vi "drive_robot.vi"(9 "steering frame velocity":dbl[](array[numeric]), 10 "starter kit differential steering frame":refnum<class "NI_Robotics_Differential Steering Frame.lvclass">, 11 "NI_Robotics_Starter Kit Host_Sim_2.0 in":refnum<class "NI_Robotics_Starter Kit Host_Sim_2.0.lvclass">) -> (3 "NI_Robotics_Starter Kit Host_Sim_2.0 out":refnum<class "NI_Robotics_Starter Kit Host_Sim_2.0.lvclass">)   [LabVIEW 2016]
uses:
  <vilib>/robotics/Starter Kit/2.0/Sim Host Interface/NI_Robotics_Starter Kit Host_Sim_2.0.lvclass
  C:/Program Files (x86)/National Instruments/LabVIEW 2016/vi.lib/robotics/Starter Kit/Host Interface/NI_Robotics_Starter Kit Host.lvclass
  <vilib>/robotics/Steering/Differential Steering Frame/NI_Robotics_Differential Steering Frame.lvclass
  C:/Program Files (x86)/National Instruments/LabVIEW 2016/vi.lib/robotics/Steering/Steering Frame/NI_Robotics_Steering Frame.lvclass
  <vilib>/robotics/Steering/Steering Frame/Apply Steering Frame Velocity to Motors.vi
  <vilib>/robotics/Steering/Steering Frame/NI_Robotics_Steering Frame.lvclass
  <vilib>/robotics/Starter Kit/Host Interface/NI_Robotics_Starter Kit Host.lvclass
  C:/Program Files (x86)/National Instruments/LabVIEW 2016/vi.lib/robotics/Steering/Special Steering Frame/NI_Robotics_Special Steering Frame.lvclass
panel:
  out "ccw motor velocity setpoints":dbl[](array[numeric])
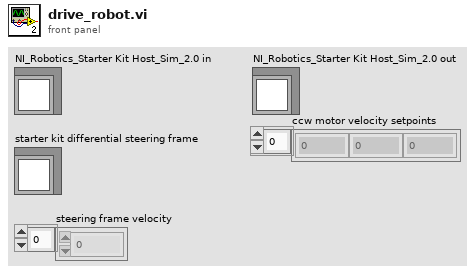
[diagram p1: front panel]
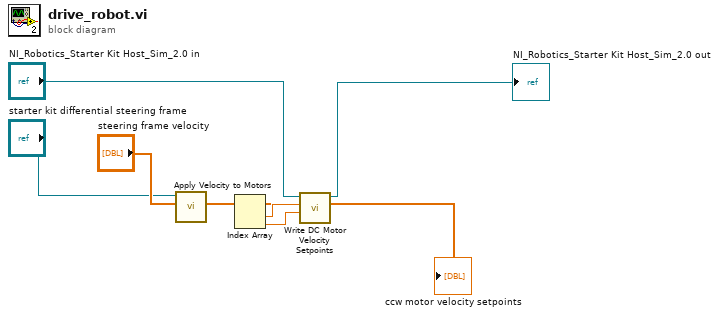
[diagram p0: block diagram]
diagram:
  n1 = call-poly <vilib>:"Apply Velocity to Motors.vi"("steering frame velocity"="steering frame velocity", "steering frame in"="starter kit differential steering frame") -> ("ccw motor velocity setpoints"=w3:dbl[])  [unwired: 5 in, 4 out]
  "ccw motor velocity setpoints" <- w3
  n2 = Index Array(array=w3) -> (element #1=w4:dbl, element #2=w5:dbl)  [unwired: 2 in]
  n3 = call <vilib>:"Write DC Motor Velocity Setpoints.vi"("right motor ccw velocity (rad/s)"=w5, "left motor ccw velocity (rad/s)"=w4, "starter kit host in"="NI_Robotics_Starter Kit Host_Sim_2.0 in") -> ("starter kit host out"=→"NI_Robotics_Starter Kit Host_Sim_2.0 out":refnum<class "NI_Robotics_Starter Kit Host_Sim_2.0.lvclass">)  [unwired: 7 in, 1 out]
